vi "未公开函数.vi"   [LabVIEW 2011]
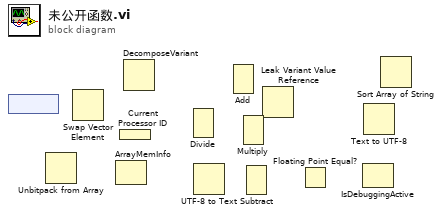
[diagram p0: block diagram]
diagram:
  n1 = node() -> ()  [unwired: 1 in, 1 out]
  n2 = Unbitpack from Array() -> ()  [unwired: 2 in, 1 out]
  n3 = Swap Vector Element() -> ()  [unwired: 3 in, 3 out]
  n4 = ArrayMemInfo() -> ()  [unwired: 7 in, 4 out]
  n5 = Current Processor ID ("当前进程ID")() -> ()  [unwired: 1 out]
  n6 = DecomposeVariant() -> ()  [unwired: 2 in, 4 out]
  n7 = Divide() -> ()  [unwired: 3 in, 2 out]
  n8 = UTF-8 to Text() -> ()  [unwired: 2 in, 2 out]
  n9 = Add() -> ()  [unwired: 3 in, 2 out]
  n10 = Multiply() -> ()  [unwired: 3 in, 2 out]
  n11 = Subtract() -> ()  [unwired: 3 in, 2 out]
  n12 = Leak Variant Value Reference() -> ()  [unwired: 2 in, 2 out]
  n13 = Floating Point Equal?() -> ()  [unwired: 3 in, 1 out]
  n14 = IsDebuggingActive() -> ()  [unwired: 10 in, 1 out]
  n15 = Text to UTF-8() -> ()  [unwired: 2 in, 2 out]
  n16 = Sort Array of String() -> ()  [unwired: 1 in, 1 out]
